vi "CameraSerialPrototype_222.vi"() -> (4 "图像时间戳":u32=16532020 format="%_32g")   [LabVIEW 2015]
uses:
  <vilib>/Instr/_visa.llb/VISA Configure Serial Port (Instr).vi
  MVCAMSDK.dll
  <vilib>/Analysis/NI_AALBase.lvlib
panel:
  in  "转动回退":bool
  in  "平移回退":bool
  in  "平移前进2":bool
  in  "平移前进1":bool
  in  "旋转前进":bool
  out "大小":i32
  out "平移信号曲线 4":cluster{"Locations":dbl[], "Amplitudes":dbl[]}[](graph)
  out "平移信号曲线 3":cluster{"Locations":dbl[], "Amplitudes":dbl[]}[](graph)
  out "实时循环时间":u32
  out "variance 3":dbl caption="纵向方差" format="%0.2f"
  out "竖直方向光强图":dbl[](graph)
  out "variance 4":dbl caption="方差" format="%0.2f"
  out "光强图 4":dbl[](graph)
  out "转动信号曲线":cluster{"Locations":dbl[], "Amplitudes":dbl[]}[](graph)
  in  "转动计数":u16
  in  "转动一次脉冲数":u16=1
  out "连接的字符串 3":string
  out "平移信号曲线 2":cluster{"Locations":dbl[], "Amplitudes":dbl[]}[](graph)
  in  "平移计数 2":u16
  in  "平移一次脉冲数 2":u16=20
  out "连接的字符串 2":string
  in  "曝光时间":i32=50
  out "平移信号曲线":cluster{"Locations":dbl[], "Amplitudes":dbl[]}[](graph)
  out "variance 2":dbl caption="方差" format="%0.2f"
  out "光强图 2":dbl[](graph)
  out "variance":dbl caption="横向方差" format="%0.2f"
  out "水平方向光强图":dbl[](graph)
  in  "平移计数":u16
  in  "平移一次脉冲数":u16=20
  out "连接的字符串":string
  in  "flow control (0:none)":u16(ring) caption="流控制（0:无）" items=["无", "XON/XOFF", "RTS/CTS", "XON/XOFF & RTS/CTS", "DTR/DSR", "XON/XOFF & DTR/DSR"]
  in  "stop bits (10: 1 bit)":u16=10 caption="停止位（10: 1位）"
  in  "奇偶 (0:none)":enum16{"None", "Odd", "Even", "Mark", "Space"}(ring) caption="奇偶（0:无）"
  in  "数据比特(默认8)":u16(ring)=8 items=["5"=5, "6"=6, "7"=7, "8"=8]
  in  "波特率(默认9600)":u32=9600
  in  "端口":refnum<visa-resource-name>="COM1"
  in  "停止":bool
  out "帧速":u32
  out "帧间耗时\n单位：（0.1ms）":u32
  out "Image":T1(plugin-control)
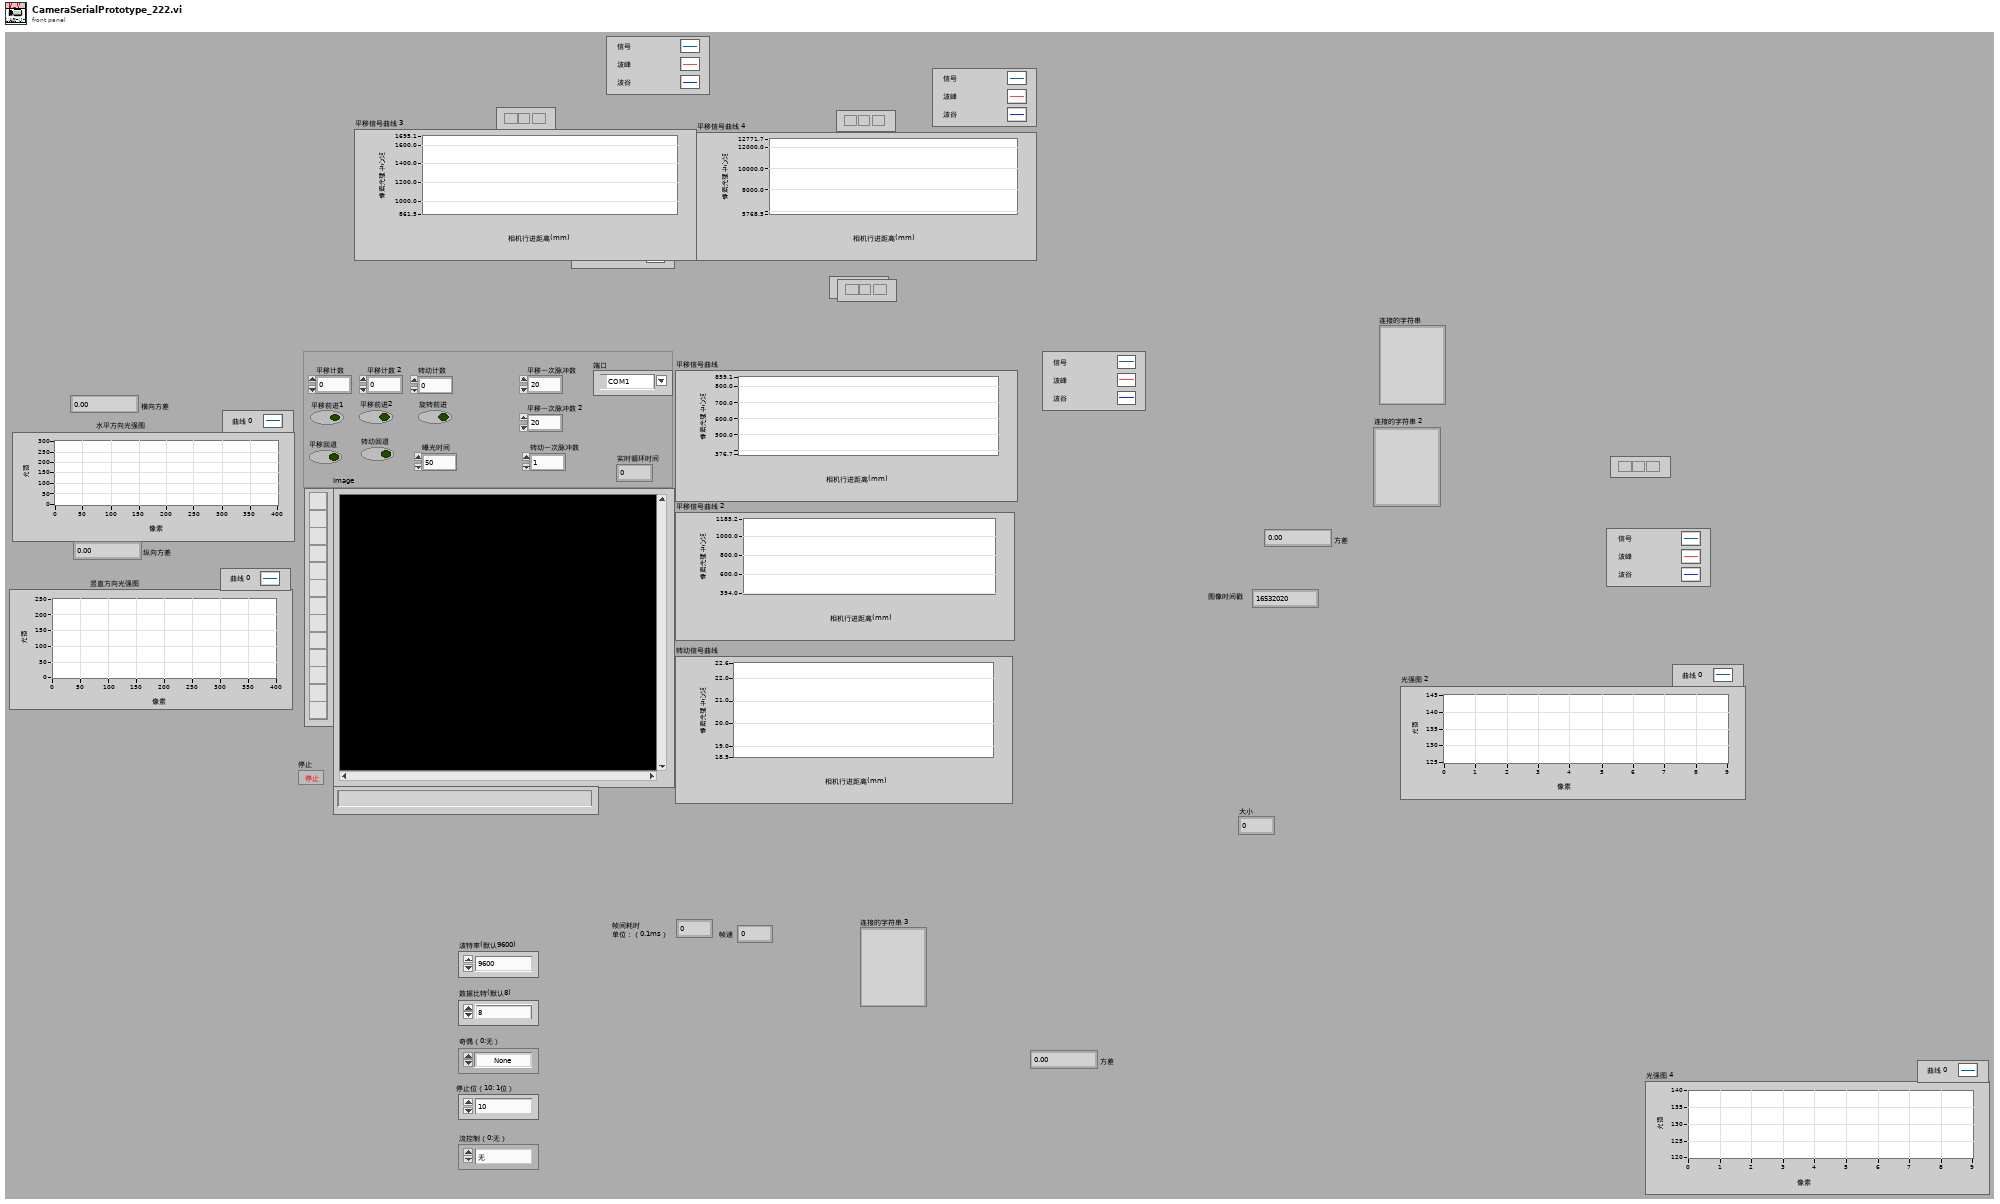
[diagram p1: front panel]
types:
  T1 = typedef "IMAQ Image.ctl" = refnum<image>
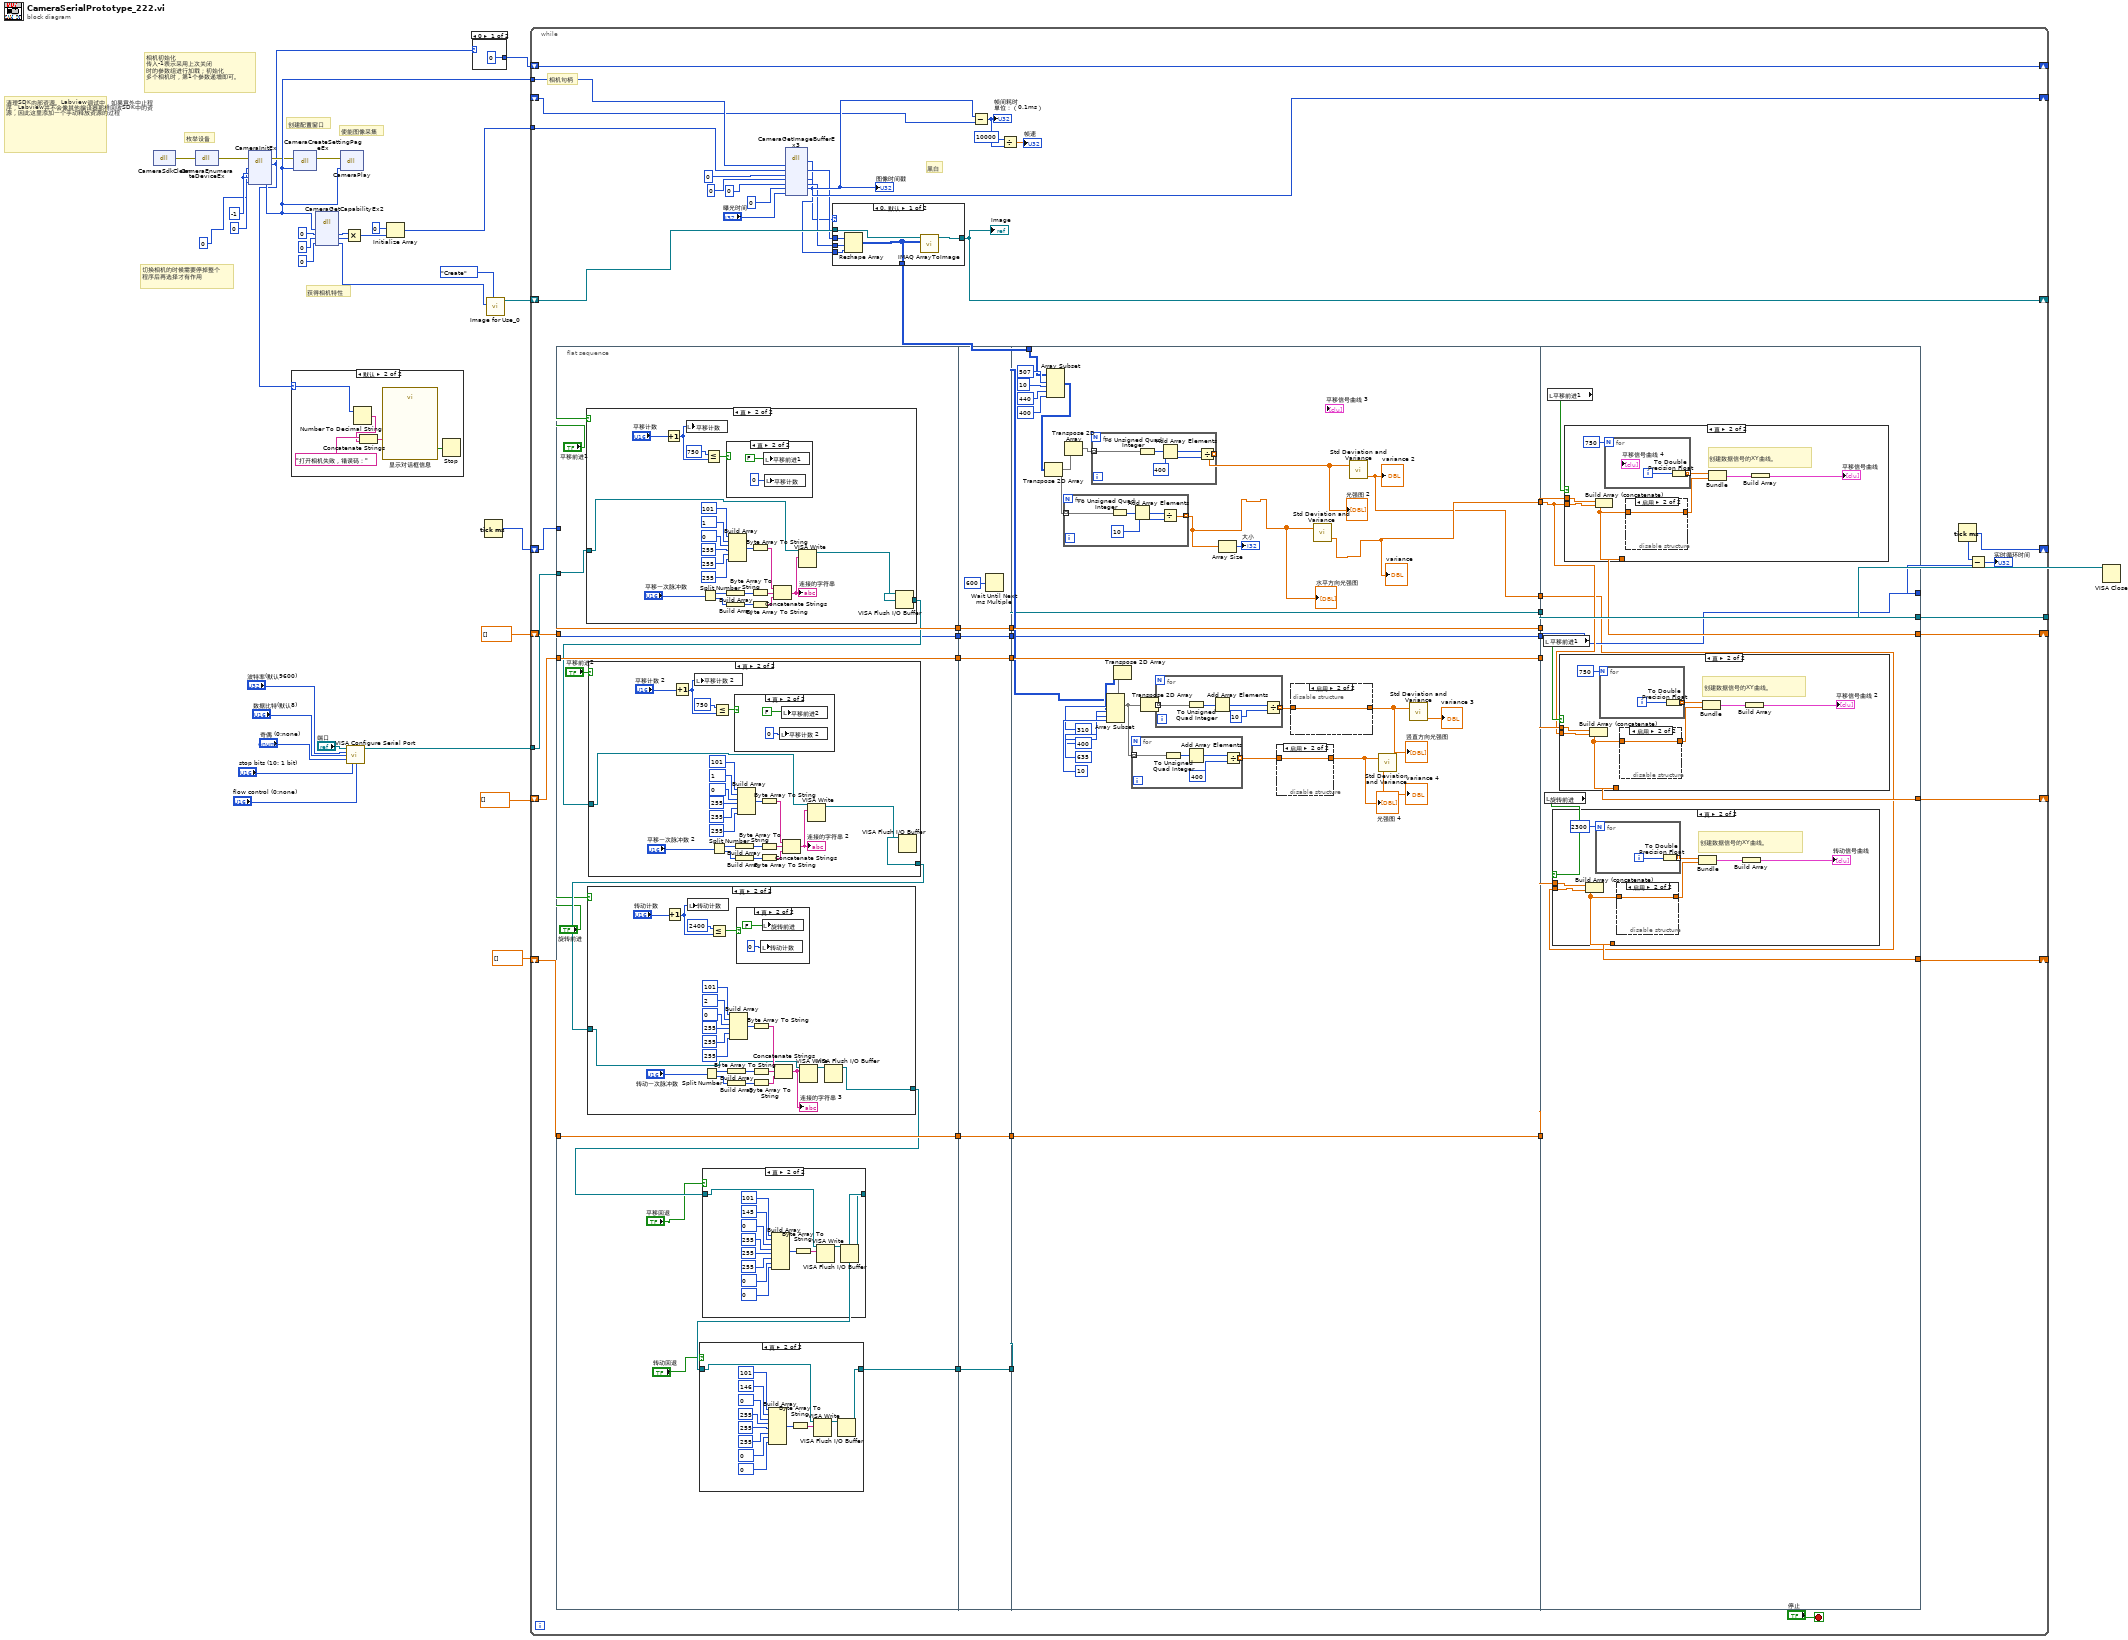
[diagram p0: block diagram]
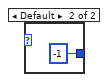
[diagram p2: hidden frame]
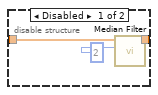
[diagram p12: hidden frame]
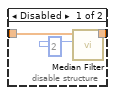
[diagram p13: hidden frame]
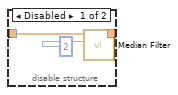
[diagram p15: hidden frame]
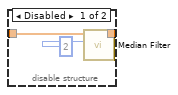
[diagram p17: hidden frame]
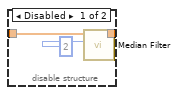
[diagram p19: hidden frame]
diagram:
  w31 = -1
  # "切换相机的时候需要停掉整个\n程序后再选择才有作用"
  # "清理SDK内部资源。Labview调试中，如果意外中止程序，Labview并不会像其他编译器那样回收SDK中的资源，因此这里添加一个手动释放资源的过程"
  # "使能图像采集"
  # "获得相机特性"
  # "创建配置窗口"
  # "相机初始化\n传入-1表示采用上次关闭\n时的参数组进行加载；初始化\n多个相机时，第1个参数递增即可。"
  # "枚举设备"
  n1 = dll-call lib="MVCAMSDK.dll" fn="CameraSdkClean"() -> (error out=w32:errorcluster)  [unwired: 4 in, 1 out]
  n2 = dll-call lib="MVCAMSDK.dll" fn="CameraEnumerateDeviceEx"(error in=w32) -> (error out=w29:errorcluster)  [unwired: 3 in, 1 out]
  n3 = dll-call lib="MVCAMSDK.dll" fn="CameraInitEx"(error in=w29, "相机索引值"=0, "参数加载方式"=w31, "要加载的参数组索引"=w31, "相机句柄"=0) -> (error out=w18:errorcluster, "返回类型"=w16:i32, "相机句柄"=w20:i32)  [unwired: 5 in, 1 out]
  n4 = case shown="默认" w16 {
    selector: w16 -> [_ w37]
    frame 0 {
    }
    frame Default {
      n5 = Number To Decimal String(number=w37) -> (decimal integer string=w34:string)  [unwired: 1 in]
      n6 = Concatenate Strings("打开相机失败，错误码：" ("字符串"), w34) -> (w36:string)
      n7 = call "显示对话框信息"("Message"=w36) -> ("结束"=w38:bool)  [unwired: 9 in, 1 out]
      n8 = Stop(stop? (T)=w38) -> ()
    }
  }
  n9 = dll-call lib="MVCAMSDK.dll" fn="CameraCreateSettingPageEx"(error in=w18, "相机句柄"=w20) -> (error out=w21:errorcluster)  [unwired: 4 in, 1 out]
  n10 = dll-call lib="MVCAMSDK.dll" fn="CameraGetCapabilityEx2"("相机句柄"=w20, "图像最大宽度"=0, "图像最大高度"=0, "是否是彩色相机(返回0:黑白;1:彩色)"=0) -> ("图像最大宽度"=w23:i32, "图像最大高度"=w22:i32, "是否是彩色相机(返回0:黑白;1:彩色)"=w14:i32)  [unwired: 5 in, 2 out]
  n11 = dll-call lib="MVCAMSDK.dll" fn="CameraPlay"(error in=w21, "相机句柄"=w20) -> ()  [unwired: 4 in, 2 out]
  n12 = Multiply(x=w23, y=w22) -> (x*y=w27:i32)
  n13 = call-poly "VISA Configure Serial Port"("VISA resource name"="端口", "baud rate (9600)"="波特率(默认9600)", "data bits (8)"="数据比特(默认8)", "parity (0:none)"="奇偶 (0:none)", "stop bits (10: 1 bit)"="stop bits (10: 1 bit)", "flow control (0:none)"="flow control (0:none)") -> ("VISA resource name out"=w6:refnum<visa-resource-name>)  [unwired: 8 in, 1 out]
  n14 = Initialize Array(0, w27) -> (w19:i32[])
  n15 = case shown="0" w16 {
    tunnel: [0 -1] -> w15
    frame 0 {
    }
    frame Default {
    }
  }
  n16 = Tick Count (ms)() -> (millisecond timer value=w1:u32)
  n17 = call "Image for Use_0.vi"("Command"=enum16{"Create", "Use", "Copy in", "Dispose"}."Create", "Image Type"=w14) -> ("Image out"=w17:T1)  [unwired: 8 in, 1 out]
  n18 = while {
    tunnel: w20 -> [w88]
    tunnel: w19 -> [w90]
    shift-right: [w87] -> _
    shift-left: w15 -> [w87]
    shift-right: [w86] -> _
    shift-left: w17 -> [w89]
    shift-right: [w85] -> _
    shift-left: _ -> [w84]
    tunnel: w6 -> [w57]
    tunnel: [w67] -> w5
    shift-right: [w64] -> _
    shift-left: dbl[] [] -> [w65]
    shift-right: [w61] -> _
    shift-left: dbl[] [] -> [w62]
    shift-right: [w59] -> _
    shift-left: dbl[] [] -> [w58]
    shift-right: [w43] -> _
    shift-left: w1 -> [w42]
    stop <- "停止" stop-if-true
    # "黑白"
    # "相机句柄"
    n19 = flat-sequence {
      tunnel: w57 -> [w105]
      tunnel: [w104] -> w56
      tunnel: w65 -> [w104]
      tunnel: [w103] -> w54
      tunnel: w62 -> [w103]
      tunnel: [w102] -> w52
      tunnel: w58 -> [w102]
      tunnel: [w97] -> w50
      tunnel: [w96] -> w46
      tunnel: w42 -> [w96]
      tunnel: w56 -> [w217]
      tunnel: [w217] -> w55
      tunnel: w54 -> [w216]
      tunnel: [w216] -> w53
      tunnel: w52 -> [w215]
      tunnel: [w215] -> w51
      tunnel: w50 -> [w214]
      tunnel: [w214] -> w49
      tunnel: [w212] -> w47
      tunnel: w46 -> [w212]
      tunnel: w70 -> [w225]
      tunnel: [w222] -> w69
      tunnel: [w224] -> w68
      tunnel: [w241] -> w66
      tunnel: w55 -> [w241]
      tunnel: [w240] -> w63
      tunnel: w53 -> [w240]
      tunnel: [w239] -> w60
      tunnel: w51 -> [w239]
      tunnel: w49 -> [w224]
      tunnel: [w223] -> w48
      tunnel: w47 -> [w223]
      tunnel: [w220] -> w41
      tunnel: w69 -> [w283]
      tunnel: w68 -> [w289]
      tunnel: [w289] -> w67
      tunnel: w66 -> [w288]
      tunnel: [w287] -> w64
      tunnel: w63 -> [w286]
      tunnel: [w284] -> w61
      tunnel: w60 -> [w282]
      tunnel: [w281] -> w59
      tunnel: [w278] -> w45
      tunnel: w48 -> [w278]
      tunnel: w41 -> [w277]
      frame #0 {
        n20 = case shown="真" "平移前进1" {
          tunnel: w105 -> [w186 w192]
          tunnel: [w186 w187] -> w101
          frame False {
          }
          frame True {
            n21 = Increment(x="平移计数") -> (x+1=w190:u16)
            n22 = local write "平移计数"(w190) -> ()
            n23 = Split Number(x="平移一次脉冲数") -> (hi(x)=w200:u8, lo(x)=w199:u8)
            n24 = Less Or Equal?(x=750, y=w190) -> (x <= y?=w202:bool)
            n25 = case shown="真" w202 {
              frame False {
              }
              frame True {
                n26 = local write "平移前进1"(FALSE) -> ()
                n27 = local write "平移计数"(u16 0 ("平移计数 2")) -> ()
              }
            }
            n28 = Build Array(w200) -> (w198:u8[])
            n29 = Build Array(w199) -> (w197:u8[])
            n30 = Build Array(101, 1, 0, 255, 255, 255) -> (w196:i32[])
            n31 = Byte Array To String(unsigned byte array=w196) -> (string=w195:string)
            n32 = Byte Array To String(unsigned byte array=w198) -> (string=w194:string)
            n33 = Byte Array To String(unsigned byte array=w197) -> (string=w193:string)
            n34 = Concatenate Strings(w195, w194, w193) -> (w189:string)
            "连接的字符串" <- w189
            n35 = VISA Write(VISA resource name=w192, write buffer=w189) -> (VISA resource name out=w188:refnum<visa-resource-name>)  [unwired: 1 in, 2 out]
            n36 = VISA Flush I/O Buffer(VISA resource name=w188) -> (VISA resource name out=w187:refnum<visa-resource-name>)  [unwired: 2 in, 1 out]
          }
        }
        n37 = case shown="真" "平移前进2" {
          tunnel: w101 -> [w160 w166]
          tunnel: [w160 w161] -> w100
          frame False {
          }
          frame True {
            n38 = Increment(x="平移计数 2") -> (x+1=w164:u16)
            n39 = local write "平移计数 2"(w164) -> ()
            n40 = Split Number(x="平移一次脉冲数 2") -> (hi(x)=w174:u8, lo(x)=w173:u8)
            n41 = Less Or Equal?(x=750, y=w164) -> (x <= y?=w176:bool)
            n42 = case shown="真" w176 {
              frame False {
              }
              frame True {
                n43 = local write "平移计数 2"(u16 0 ("平移计数 2")) -> ()
                n44 = local write "平移前进2"(FALSE) -> ()
              }
            }
            n45 = Build Array(w174) -> (w172:u8[])
            n46 = Build Array(w173) -> (w171:u8[])
            n47 = Build Array(101, 1, 0, 255, 255, 255) -> (w170:i32[])
            n48 = Byte Array To String(unsigned byte array=w170) -> (string=w169:string)
            n49 = Byte Array To String(unsigned byte array=w172) -> (string=w168:string)
            n50 = Byte Array To String(unsigned byte array=w171) -> (string=w167:string)
            n51 = Concatenate Strings(w169, w168, w167) -> (w163:string)
            "连接的字符串 2" <- w163
            n52 = VISA Write(VISA resource name=w166, write buffer=w163) -> (VISA resource name out=w162:refnum<visa-resource-name>)  [unwired: 1 in, 2 out]
            n53 = VISA Flush I/O Buffer(VISA resource name=w162) -> (VISA resource name out=w161:refnum<visa-resource-name>)  [unwired: 2 in, 1 out]
          }
        }
        n54 = case shown="真" "旋转前进" {
          tunnel: w100 -> [w134 w140]
          tunnel: [w134 w135] -> w99
          frame False {
          }
          frame True {
            n55 = Increment(x="转动计数") -> (x+1=w138:u16)
            n56 = local write "转动计数"(w138) -> ()
            n57 = Split Number(x="转动一次脉冲数") -> (hi(x)=w148:u8, lo(x)=w147:u8)
            n58 = Less Or Equal?(x=2400, y=w138) -> (x <= y?=w150:bool)
            n59 = Build Array(w148) -> (w146:u8[])
            n60 = Build Array(w147) -> (w145:u8[])
            n61 = Build Array(101, 2, 0, 255, 255, 255) -> (w144:i32[])
            n62 = case shown="真" w150 {
              frame False {
              }
              frame True {
                n63 = local write "转动计数"(u16 0 ("平移计数 2")) -> ()
                n64 = local write "旋转前进"(FALSE) -> ()
              }
            }
            n65 = Byte Array To String(unsigned byte array=w144) -> (string=w143:string)
            n66 = Byte Array To String(unsigned byte array=w146) -> (string=w142:string)
            n67 = Byte Array To String(unsigned byte array=w145) -> (string=w141:string)
            n68 = Concatenate Strings(w143, w142, w141) -> (w137:string)
            "连接的字符串 3" <- w137
            n69 = VISA Write(VISA resource name=w140, write buffer=w137) -> (VISA resource name out=w136:refnum<visa-resource-name>)  [unwired: 1 in, 2 out]
            n70 = VISA Flush I/O Buffer(VISA resource name=w136) -> (VISA resource name out=w135:refnum<visa-resource-name>)  [unwired: 2 in, 1 out]
          }
        }
        n71 = case shown="真" "平移回退" {
          tunnel: w99 -> [w120 w126]
          tunnel: [w120 w121] -> w98
          frame False {
          }
          frame True {
            n72 = Build Array(101, 145, 0, 255, 255, 255, 0, 0) -> (w127:i32[])
            n73 = Byte Array To String(unsigned byte array=w127) -> (string=w125:string)
            n74 = VISA Write(VISA resource name=w126, write buffer=w125) -> (VISA resource name out=w122:refnum<visa-resource-name>)  [unwired: 1 in, 2 out]
            n75 = VISA Flush I/O Buffer(VISA resource name=w122) -> (VISA resource name out=w121:refnum<visa-resource-name>)  [unwired: 2 in, 1 out]
          }
        }
        n76 = case shown="真" "转动回退" {
          tunnel: w98 -> [w106 w112]
          tunnel: [w106 w107] -> w97
          frame False {
          }
          frame True {
            n77 = Build Array(101, 146, 0, 255, 255, 255, 0, 0) -> (w113:i32[])
            n78 = Byte Array To String(unsigned byte array=w113) -> (string=w111:string)
            n79 = VISA Write(VISA resource name=w112, write buffer=w111) -> (VISA resource name out=w108:refnum<visa-resource-name>)  [unwired: 1 in, 2 out]
            n80 = VISA Flush I/O Buffer(VISA resource name=w108) -> (VISA resource name out=w107:refnum<visa-resource-name>)  [unwired: 2 in, 1 out]
          }
        }
      }
      frame #1 {
        n81 = Wait Until Next ms Multiple(millisecond multiple=u32 600 ("毫秒倍数")) -> ()  [unwired: 1 out]
      }
      frame #2 {
        n82 = Array Subset(array=w225, index (row)=507 ("索引"), length (row)=10 ("长度"), index (col)=440 ("长度"), length (col)=400 ("索引")) -> (w244:u8[][])
        n83 = Transpose 2D Array(2D array=w244) -> (transposed array=w242:u8[][])
        n84 = for {
          tunnel: w242 -> [w275] mode=indexing
          tunnel: [w273] -> w218 mode=indexing
          n85 = To Unsigned Quad Integer(1:w275) -> (0:w274:u64[])
          n86 = Add Array Elements(numeric array=w274) -> (sum=w276:u64)
          n87 = Divide(x=w276, y=u64 10) -> (x/y=w273:dbl)
        }
        "水平方向光强图" <- w218
        n88 = Transpose 2D Array(2D array=w242) -> (transposed array=w243:u8[][])
        n89 = for {
          tunnel: w243 -> [w270] mode=indexing
          tunnel: [w268] -> w221 mode=indexing
          n90 = To Unsigned Quad Integer(1:w270) -> (0:w269:u64[])
          n91 = Add Array Elements(numeric array=w269) -> (sum=w271:u64)
          n92 = Divide(x=w271, y=u64 400) -> (x/y=w268:dbl)
        }
        "光强图 2" <- w221
        n93 = Array Subset(array=w225, index (row)=310 ("索引"), length (row)=400 ("长度"), index (col)=635 ("长度"), length (col)=10 ("索引")) -> (w228:u8[][])
        n94 = Transpose 2D Array(2D array=w228) -> (transposed array=w227:u8[][])
        n95 = for {
          tunnel: w227 -> [w261] mode=indexing
          tunnel: [w259] -> w230 mode=indexing
          n96 = To Unsigned Quad Integer(1:w261) -> (0:w260:u64[])
          n97 = Add Array Elements(numeric array=w260) -> (sum=w262:u64)
          n98 = Divide(x=w262, y=u64 400) -> (x/y=w259:dbl)
        }
        n99 = Transpose 2D Array(2D array=w227) -> (transposed array=w232:u8[][])
        n100 = for {
          tunnel: w232 -> [w252] mode=indexing
          tunnel: [w250] -> w231 mode=indexing
          n101 = To Unsigned Quad Integer(1:w252) -> (0:w251:u64[])
          n102 = Add Array Elements(numeric array=w251) -> (sum=w253:u64)
          n103 = Divide(x=w253, y=u64 10) -> (x/y=w250:dbl)
        }
        n104 = Array Size(array=w218) -> (size(s)=→"大小":i32)
        n105 = disable-structure shown="启用" {
          disable-tunnel: w230 -> [w265 w266]
          disable-tunnel: [w263 w266] -> w233
          frame Disabled {
            n106 = call <vilib>:"Median Filter.vi"("left rank"=2, "X"=w265) -> ("Filtered X"=w263:dbl[])  [unwired: 8 in, 1 out]
          }
          frame Enabled {
          }
        }
        "光强图 4" <- w233
        n107 = disable-structure shown="启用" {
          disable-tunnel: w231 -> [w256 w257]
          disable-tunnel: [w254 w257] -> w234
          frame Disabled {
            n108 = call <vilib>:"Median Filter.vi"("left rank"=2, "X"=w256) -> ("Filtered X"=w254:dbl[])  [unwired: 8 in, 1 out]
          }
          frame Enabled {
          }
        }
        "竖直方向光强图" <- w234
        n109 = call <vilib>:"Std Deviation and Variance.vi"("X"=w218) -> ("variance"=w222:dbl)  [unwired: 1 in, 2 out]
        "variance" <- w222
        n110 = call <vilib>:"Std Deviation and Variance.vi"("X"=w221) -> ("variance"=w220:dbl)  [unwired: 1 in, 2 out]
        "variance 2" <- w220
        n111 = call <vilib>:"Std Deviation and Variance.vi"("X"=w233) -> ("variance"=→"variance 4":dbl)  [unwired: 1 in, 2 out]
        n112 = call <vilib>:"Std Deviation and Variance.vi"("X"=w234) -> ("variance"=→"variance 3":dbl)  [unwired: 1 in, 2 out]
      }
      frame #3 {
        n113 = local read "平移前进1"() -> (w285:bool)
        n114 = local read "旋转前进"() -> (w280:bool)
        n115 = local read "平移前进1"() -> (w279:bool)
        n116 = case shown="真" w280 {
          tunnel: w282 -> [w290 w292]
          tunnel: w277 -> [_ w293]
          tunnel: [w290 w291] -> w281
          frame False {
          }
          frame True {
            # "创建数据信号的XY曲线。"
            n117 = Build Array (concatenate)(w292, w293) -> (w291:dbl[])
            n118 = for {
              N: i64 2300 ("数值") -> [_]
              tunnel: [w299] -> w297 mode=indexing
              i -> [w300]
              n119 = To Double Precision Float(number=w300) -> (double precision float=w299:dbl)
            }
            n120 = disable-structure shown="启用" {
              disable-tunnel: w291 -> [w302 w304]
              disable-tunnel: [w301 w304] -> w296
              frame Disabled {
                n121 = call <vilib>:"Median Filter.vi"("left rank"=2, "X"=w302) -> ("Filtered X"=w301:dbl[])  [unwired: 8 in, 1 out]
              }
              frame Enabled {
              }
            }
            n122 = Bundle(w297, w296) -> (w294:cluster{dbl[], dbl[]})  [unwired: 1 in]
            n123 = Build Array(w294) -> (→"转动信号曲线":cluster{dbl[], dbl[]}[])
          }
        }
        n124 = case shown="真" w285 {
          tunnel: w286 -> [w305 w307]
          tunnel: w283 -> [_ w308]
          tunnel: [w305 w306] -> w284
          frame False {
          }
          frame True {
            # "创建数据信号的XY曲线。"
            n125 = Build Array (concatenate)(w307, w308) -> (w306:dbl[])
            n126 = for {
              N: i64 750 ("数值") -> [_]
              tunnel: [w314] -> w312 mode=indexing
              i -> [w315]
              n127 = To Double Precision Float(number=w315) -> (double precision float=w314:dbl)
            }
            n128 = disable-structure shown="启用" {
              disable-tunnel: w306 -> [w317 w319]
              disable-tunnel: [w316 w319] -> w311
              frame Disabled {
                n129 = call <vilib>:"Median Filter.vi"("left rank"=2, "X"=w317) -> ("Filtered X"=w316:dbl[])  [unwired: 8 in, 1 out]
              }
              frame Enabled {
              }
            }
            n130 = Bundle(w312, w311) -> (w309:cluster{dbl[], dbl[]})  [unwired: 1 in]
            n131 = Build Array(w309) -> (→"平移信号曲线 2":cluster{dbl[], dbl[]}[])
          }
        }
        n132 = case shown="真" w279 {
          tunnel: w288 -> [w320 w322]
          tunnel: w283 -> [_ w323]
          tunnel: [w320 w321] -> w287
          frame False {
          }
          frame True {
            # "创建数据信号的XY曲线。"
            n133 = Build Array (concatenate)(w322, w323) -> (w321:dbl[])
            n134 = for {
              N: i64 750 ("数值") -> [_]
              tunnel: [w329] -> w327 mode=indexing
              i -> [w330]
              n135 = To Double Precision Float(number=w330) -> (double precision float=w329:dbl)
            }
            n136 = disable-structure shown="启用" {
              disable-tunnel: w321 -> [w332 w334]
              disable-tunnel: [w331 w334] -> w326
              frame Disabled {
                n137 = call <vilib>:"Median Filter.vi"("left rank"=2, "X"=w332) -> ("Filtered X"=w331:dbl[])  [unwired: 8 in, 1 out]
              }
              frame Enabled {
              }
            }
            n138 = Bundle(w327, w326) -> (w324:cluster{dbl[], dbl[]})  [unwired: 1 in]
            n139 = Build Array(w324) -> (→"平移信号曲线":cluster{dbl[], dbl[]}[])
          }
        }
      }
    }
    n140 = dll-call lib="MVCAMSDK.dll" fn="CameraGetImageBufferEx3"("相机句柄"=w88, "图像数据缓冲区"=w90, "图像输出格式(0:8位灰度;1:24位彩色;2:32位彩色，3：BGR24彩色 4：BGRA32位彩色)"=0, "图像宽度"=0, "图像高度"=0, "时间戳(单位为100微秒)"=0, "抓图超时时间(毫秒)"="曝光时间") -> ("返回类型"=w72:i32, "图像数据缓冲区"=w75:u8[], "图像宽度"=w73:i32, "图像高度"=w74:i32, "时间戳(单位为100微秒)"=w85:u32)  [unwired: 6 in, 2 out]
    "图像时间戳" <- w85
    n141 = case shown="0, 默认" w72 {
      tunnel: w75 -> [w340 _]
      tunnel: w89 -> [w337 w341]
      tunnel: w74 -> [w339 _]
      tunnel: w73 -> [w338 _]
      tunnel: [w336 w341] -> w86
      tunnel: [w335 _] -> w70
      frame 0, Default {
        n142 = Reshape Array(w340, w339, w338) -> (w335:u8[][])
        n143 = call "IMAQ ArrayToImage"("Image Pixels (U8)"=w335, "Image"=w337) -> ("Image Out"=w336:T1)  [unwired: 8 in, 1 out]
      }
      frame -12 {
      }
    }
    "Image" <- w86
    n144 = Subtract(x=w85, y=w84) -> (x-y=w83:u32)
    "帧间耗时\n单位：（0.1ms）" <- w83
    n145 = Divide(x=u32 10000 ("帧间耗时"), y=w83) -> (x/y=→"帧速":dbl)
    n146 = Tick Count (ms)() -> (millisecond timer value=w43:u32)
    n147 = Subtract(x=w43, y=w45) -> (x-y=→"实时循环时间":u32)
  }
  n148 = VISA Close(VISA resource name=w5) -> ()  [unwired: 1 in, 1 out]
